vi "test.InvokeModuleReference.vi"() -> ()   [LabVIEW 2014]
uses:
  Private/Class/class.GLue.lvclass/class.GLue.ctl
  <vilib>/Utility/semaphor.llb/Acquire Semaphore.vi
  Private/Class/meth.RunChunk.vi
  <vilib>/Utility/semaphor.llb/Release Semaphore.vi
  Private/Class/class.GLue.lvclass
panel:
  out "data":string[](array[string])
  out "error out 2":errorcluster
  out "error out":errorcluster
  out "Return":variant
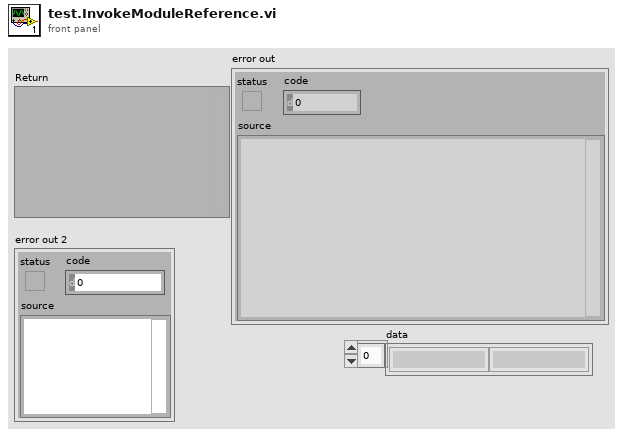
[diagram p1: front panel]
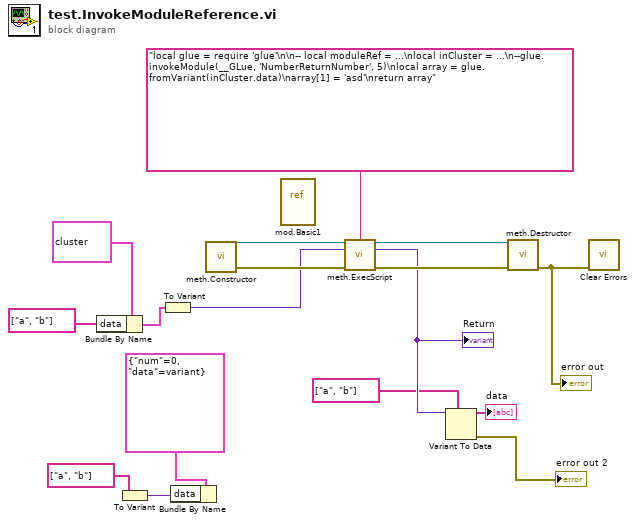
[diagram p0: block diagram]
diagram:
  n1 = Bundle By Name(cluster=cluster{"data":variant, "num":i32} {"data"=variant, "num"=0}, "data"=string[] ["a", "b"]) -> (w5:cluster{"data":variant, "num":i32})
  n2 = To Variant(anything=string[] ["a", "b"]) -> (Variant=w7:variant)
  n3 = To Variant(anything=w5) -> (Variant=w1:variant)
  n4 = Bundle By Name(cluster=cluster{"num":i32, "data":variant} {"num"=0, "data"=variant}, "data"=w7) -> ()  [unwired: 1 out]
  n5 = call "meth.Constructor.vi"() -> ("GLue out"=w14:refnum<class "class.GLue.lvclass">, "error out"=w17:errorcluster)  [unwired: 14 in]
  n6 = vi-ref "mod.Basic1.vi"() -> ()  [unwired: 1 out]
  n7 = call "meth.ExecScript.vi"("GLue in"=w14, "Script"="local glue = require 'glue'\n\n-- local moduleRef = ...\nlocal inCluster = ...\n--glue.invokeModule(__GLue, 'NumberReturnNumber', 5)\nlocal array = glue.fromVariant(inCluster.data)\narray[1] = 'asd'\nreturn array", "Argument"=w1, "error in"=w17) -> ("GLue out"=w15:refnum<class "class.GLue.lvclass">, "Return"=w10:variant, "error out"=w16:errorcluster)  [unwired: 9 in]
  "Return" <- w10
  n8 = Variant To Data(type=string[] ["a", "b"], Variant=w10) -> (data=→"data":string[], error out=→"error out 2":errorcluster)  [unwired: 1 in]
  n9 = call "meth.Destructor.vi"("GLue in"=w15, "error in"=w16) -> ("error out"=w13:errorcluster)  [unwired: 13 in]
  "error out" <- w13
  n10 = call <vilib>:"Clear Errors.vi"("error in (no error)"=w13) -> ()  [unwired: 5 in, 2 out]
